vi "Write setup configuration.vi"(8 "error in (no error)":errorcluster, 11 "Channel in":refnum<class "Channel.lvclass">) -> (0 "error out":errorcluster, 3 "Channel out":refnum<class "Channel.lvclass">)   [LabVIEW 2018, in "Channel.lvclass"]
uses:
  Channel.lvclass
  Channel.lvclass/Channel.ctl
  Sim_CCD/Sim_CCD.lvclass/Sim_CCD.ctl
  Sim_CCD/Sim_CCD.lvclass
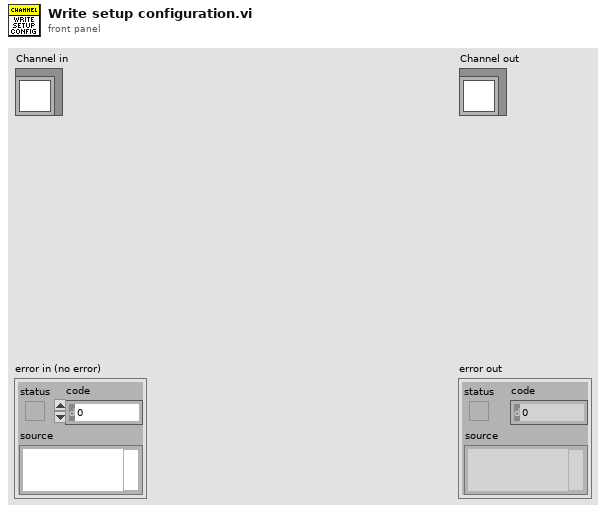
[diagram p1: front panel]
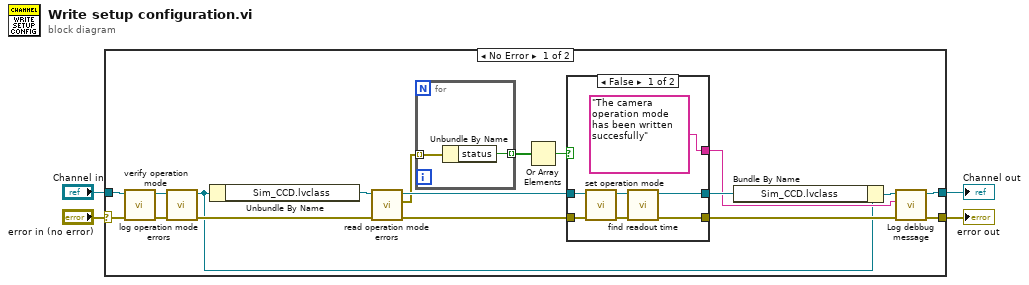
[diagram p0: block diagram]
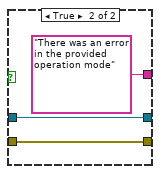
[diagram p2: hidden frame]
diagram:
  n1 = case shown="No Error" "error in (no error)" {
    selector: "error in (no error)" -> [w20 w36]
    tunnel: [w12 w36] -> w3
    tunnel: [w13 w35] -> w1
    tunnel: "Channel in" -> [w21 w35]
    frame No Error {
      n2 = call-dynamic "verify operation mode.vi"("error in (no error)"=w20, "Channel in"=w21) -> ("error out"=w7:errorcluster, "Channel out"=w8:refnum<class "Channel.lvclass">)  [unwired: 8 in]
      n3 = call "log operation mode errors.vi"("error in (no error)"=w7, "Channel in"=w8) -> ("error out"=w6:errorcluster, "Channel out"=w5:refnum<class "Channel.lvclass">)  [unwired: 8 in]
      n4 = Unbundle By Name(w5) -> ("Sim_CCD.lvclass"=w19:refnum<class "Sim_CCD.lvclass">)
      n5 = call "read operation mode errors.vi"("error in (no error)"=w6, "Simulated_CCD_Camera in"=w19) -> ("error out"=w18:errorcluster, "WRITE SETUP errors"=w16:errorcluster[], "Simulated_CCD_Camera out"=w17:refnum<class "Sim_CCD.lvclass">)  [unwired: 7 in]
      n6 = for {
        tunnel: w16 -> [w24] mode=indexing
        tunnel: [w23] -> w15 mode=indexing
        n7 = Unbundle By Name(w24) -> ("status"=w23:bool)
      }
      n8 = Or Array Elements(Boolean array=w15) -> (logical OR=w14:bool)
      n9 = case shown="False" w14 {
        tunnel: w17 -> [w31 w34]
        tunnel: w18 -> [w30 w33]
        tunnel: [w28 w33] -> w11
        tunnel: [w27 w34] -> w22
        tunnel: ["The camera operation mode has been written succesfully" ("String") "There was an error in the provided operation mode" ("String")] -> w9
        frame False {
          n10 = call-dynamic "set operation mode.vi"("error in (no error)"=w30, "CCDCamera in"=w31) -> ("error out"=w29:errorcluster, "CCDCamera out"=w26:refnum<class "Sim_CCD.lvclass">)  [unwired: 8 in]
          n11 = call-dynamic "find readout time.vi"("error in (no error)"=w29, "Simulated_CCD_Camera in"=w26) -> ("error out"=w28:errorcluster, "Simulated_CCD_Camera out"=w27:refnum<class "Sim_CCD.lvclass">)  [unwired: 8 in]
        }
        frame True {
        }
      }
      n12 = Bundle By Name(cluster=w5, "Sim_CCD.lvclass"=w22) -> (w10:refnum<class "Channel.lvclass">)
      n13 = call "Log debbug message.vi"("error in (no error)"=w11, "String"=w9, "Channel in"=w10) -> ("error out"=w12:errorcluster, "Channel out"=w13:refnum<class "Channel.lvclass">)  [unwired: 7 in]
    }
    frame Error {
    }
  }
  "error out" <- w3
  "Channel out" <- w1
